vi "Query.vi"(8 "error in (no error)":errorcluster, 9 "Data":i32, 10 "Command":string, 11 "Port In":refnum<visa-resource-name>="COM14") -> (0 "error out":errorcluster, 1 "Reply Float":dbl, 2 "Reply Int":u32, 3 "Port Out":refnum<visa-resource-name>="COM14", 4 "CRC ok?":bool)   [LabVIEW 2023, in "Temperature Controller.lvlib"]
uses:
  Temperature Controller.lvlib
panel:
  out "all lower case string":string
  out "read buffer":string
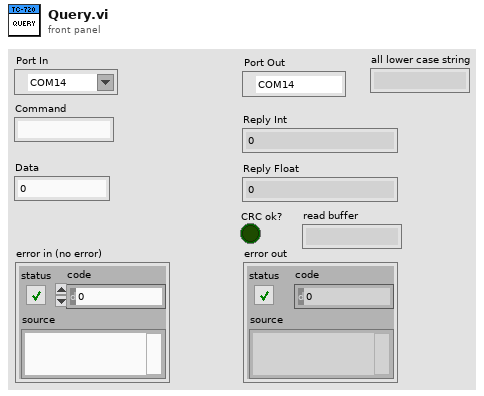
[diagram p1: front panel]
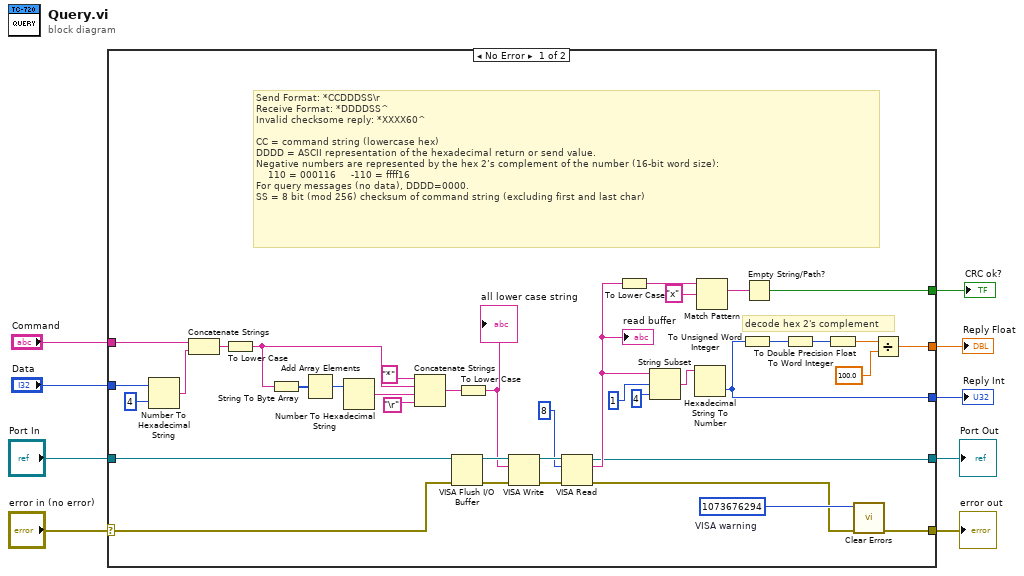
[diagram p0: block diagram]
diagram:
  n1 = case shown="No Error" "error in (no error)" {
    selector: "error in (no error)" -> [w45 w48]
    tunnel: [w25 w48] -> w8
    tunnel: "Port In" -> [w44 w49]
    tunnel: [w17 w49] -> w6
    tunnel: [w21 _] -> w3
    tunnel: "Command" -> [w14 _]
    tunnel: [w26 _] -> w4
    tunnel: [w23 _] -> w2
    tunnel: "Data" -> [w15 _]
    frame No Error {
      w24 = 1073676294  # VISA warning
      # "decode hex 2's complement"
      # "Send Format: *CCDDDSS\\r\nReceive Format: *DDDDSS^\nInvalid checksome reply: *XXXX60^\n\nCC = command string (lowercase hex)\nDDDD = ASCII representation of the hexadecimal return or send value.\nNegative numbers are represented by the hex 2’s complement of the number (16-bit word size):\n    110 = 000116     -110 = ffff16\nFor query messages (no data), DDDD=0000.\nSS = 8 bit (mod 256) checksum of command string (excluding first and last char)"
      n2 = Number To Hexadecimal String(1:i16 4 ("width (-)"), 2:w15) -> (0:w13:string)
      n3 = Concatenate Strings(w14, w13) -> (w11:string)
      n4 = To Lower Case(string=w11) -> (all lower case string=w10:string)
      n5 = String To Byte Array(string=w10) -> (unsigned byte array=w40:u8[])
      n6 = Add Array Elements(numeric array=w40) -> (sum=w39:u8)
      n7 = Number To Hexadecimal String(2:w39) -> (0:w38:string)  [unwired: 1 out]
      n8 = Concatenate Strings("*" ("Substring"), w10, w38, "\r") -> (w36:string)
      n9 = VISA Flush I/O Buffer(VISA resource name=w44, error in (no error)=w45) -> (VISA resource name out=w43:refnum<visa-resource-name>, error out=w46:errorcluster)  [unwired: 1 out]
      n10 = To Lower Case(string=w36) -> (all lower case string=w35:string)
      "all lower case string" <- w35
      n11 = VISA Write(VISA resource name=w43, write buffer=w35, error in (no error)=w46) -> (VISA resource name out=w42:refnum<visa-resource-name>, error out=w47:errorcluster)  [unwired: 1 out]
      n12 = VISA Read(VISA resource name=w42, byte count=u32 8, error in (no error)=w47) -> (VISA resource name out=w17:refnum<visa-resource-name>, read buffer=w28:string, error out=w16:errorcluster)  [unwired: 1 out]
      "read buffer" <- w28
      n13 = To Lower Case(string=w28) -> (all lower case string=w33:string)
      n14 = String Subset(string=w28, offset (0)=1, length (rest)=4 ("length (rest)")) -> (substring=w29:string)
      n15 = Hexadecimal String To Number(string=w29) -> (number=w21:u32)  [unwired: 3 out]
      n16 = Match Pattern(string=w33, regular expression="x") -> (match substring=w31:string)  [unwired: 4 out]
      n17 = To Unsigned Word Integer(number=w21) -> (unsigned 16bit integer=w20:u16)
      n18 = Empty String/Path?(string/path=w31) -> (empty?=w26:bool)
      n19 = To Word Integer(number=w20) -> (16bit integer=w19:i16)
      n20 = To Double Precision Float(number=w19) -> (double precision float=w18:dbl)
      n21 = call <vilib>:"Clear Errors.vi"("error in (no error)"=w16, "specific error code to clear (0: all)"=w24) -> ("error out"=w25:errorcluster)  [unwired: 4 in, 1 out]
      n22 = Divide(x=w18, y=100.0) -> (x/y=w23:dbl)
    }
    frame Error {
    }
  }
  "Port Out" <- w6
  "error out" <- w8
  "CRC ok?" <- w4
  "Reply Int" <- w3
  "Reply Float" <- w2
